vi "OPEN.vi"(11 "Pump_1AI_1DO_2DI in":refnum<class "ValveModbus.lvclass">) -> (3 "Pump_1AI_1DO_2DI out":refnum<class "ValveModbus.lvclass">)   [LabVIEW 2019, in "ValveModbus.lvclass"]
uses:
  ValveModbus.lvclass
  ValveModbus.lvclass/ValveModbus.ctl
  TypeDef/StateValveModbus.ctl
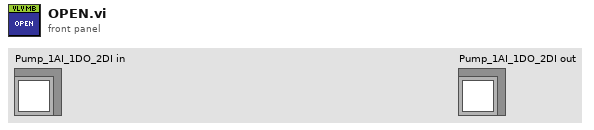
[diagram p1: front panel]
types:
  T1 = typedef "StateValveModbus.ctl" = enum16{"IDLE", "OPEN", "CLOSE", "OPENING", "CLOSING", "STOP"}
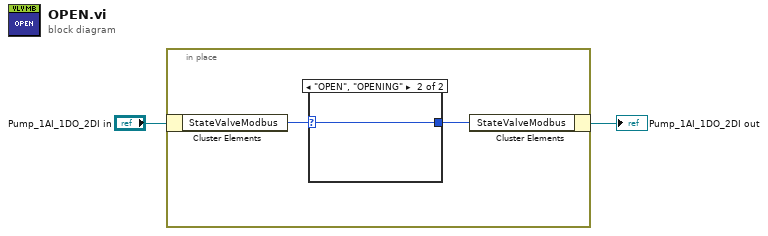
[diagram p0: block diagram]
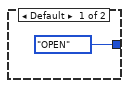
[diagram p2: hidden frame]
diagram:
  n1 = in-place {
    n2 = in-place-cluster #1("Pump_1AI_1DO_2DI in") -> ("StateValveModbus"=w4:T1)
    n3 = case shown="\"OPEN\", \"OPENING\"" w4 {
      selector: w4 -> [_ w6]
      tunnel: [StateValveModbus."OPEN" ("StateValveModbus") w6] -> w3
      frame Default {
      }
      frame "OPEN", "OPENING" {
      }
    }
    n4 = in-place-cluster #1("StateValveModbus"=w3) -> (→"Pump_1AI_1DO_2DI out":refnum<class "ValveModbus.lvclass">)
  }
